vi "Write Result.vi"(8 "error in (no error)":errorcluster, 10 "Acquired Result.lvclass":refnum<class "Acquired Result.lvclass">, 11 "Result Reply Msg in":refnum<class "Result Reply Msg.lvclass">) -> (0 "error out":errorcluster, 3 "Result Reply Msg out":refnum<class "Result Reply Msg.lvclass">)   [LabVIEW 2015, in "Result Reply Msg.lvclass"]
uses:
  Result Reply Msg.lvclass
  Results/Acquired Result/Acquired Result.lvclass
  Result Reply Msg.lvclass/Result Reply Msg.ctl
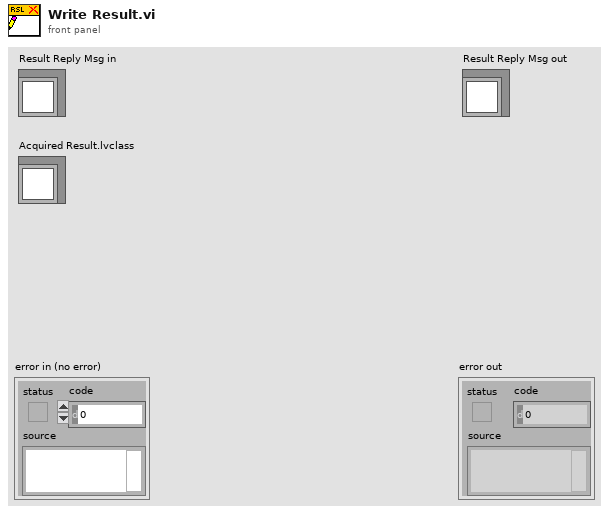
[diagram p1: front panel]
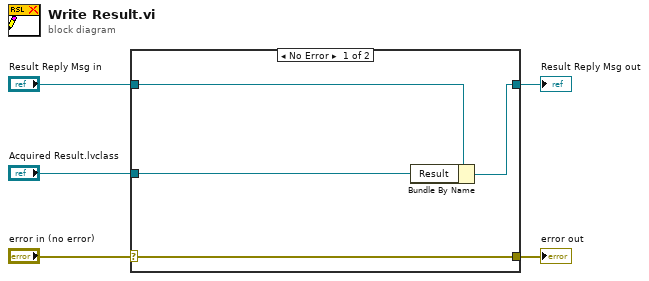
[diagram p0: block diagram]
diagram:
  n1 = case shown="No Error" "error in (no error)" {
    selector: "error in (no error)" -> [w9 w10]
    tunnel: [w9 w10] -> w4
    tunnel: [w7 w11] -> w2
    tunnel: "Result Reply Msg in" -> [w8 w11]
    tunnel: "Acquired Result.lvclass" -> [w6 _]
    frame No Error {
      n2 = Bundle By Name(cluster=w8, "Result"=w6) -> (w7:refnum<class "Result Reply Msg.lvclass">)
    }
    frame Error {
    }
  }
  "error out" <- w4
  "Result Reply Msg out" <- w2
